vi "Format Test Configurations.vi"(0 "Test Configuration":T3(array[cluster]) {"Test Ranking" items=["Low", "Normal", "High"]}) -> (4 "formatted string":string)   [LabVIEW 2020]
uses:
  <vilib>/addons/analyzer/_analyzerctrls.llb/VIAnCtl TestRanking.ctl
  <vilib>/addons/analyzer/_analyzerctrls.llb/VIAnCtl Config Control Value.ctl
  <vilib>/Utility/sysdir.llb/System Directory Type.ctl
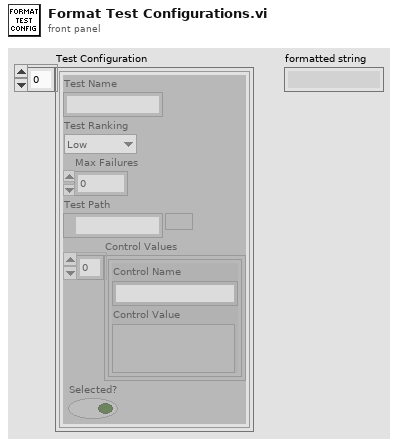
[diagram p1: front panel]
types:
  T1 = typedef "VIAnCtl TestRanking.ctl" = u16
  T2 = typedef "VIAnCtl Config Control Value.ctl" = cluster{"Control Name":string, "Control Value":variant}
  T3 = cluster{"Test Name":string, "Test Ranking":T1, "Max Failures":u32, "Test Path":path, "Control Values":T2[], "Selected?":bool}[]
  T4 = typedef "System Directory Type.ctl" = i32
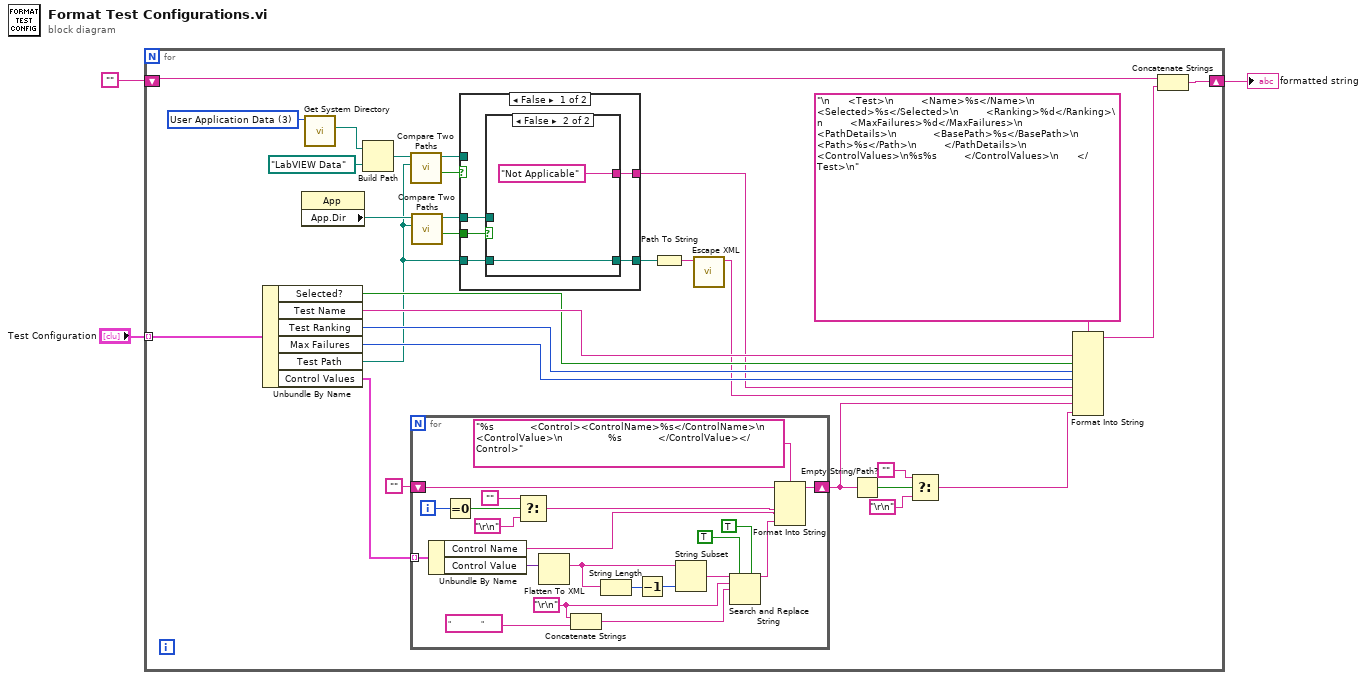
[diagram p0: block diagram]
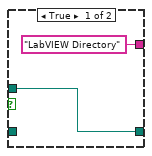
[diagram p2: hidden frame]
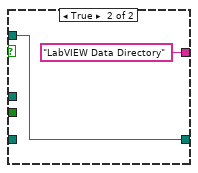
[diagram p3: hidden frame]
diagram:
  n1 = for {
    tunnel: "Test Configuration" -> [w33] mode=indexing
    shift-right: [w31] -> w1
    shift-left: "" -> [w32]
    w10 = T4 3 items=["User Home"=0, "User Desktop"=1, "User Documents"=2, "User Application Data"=3, "User Preferences"=4, "User Temporary"=5, "Public Documents"=6, "Public Application Data"=7, "Public Preferences"=8, "Public Cache"=13, "System Core Libraries"=9, "System Installed Libraries"=10, "Application Files"=11, "Boot Volume Root"=12] ("system directory type")
    n2 = Unbundle By Name(w33) -> ("Selected?"=w24:bool, "Test Name"=w30:string, "Test Ranking"=w28:T1, "Max Failures"=w27:u32, "Test Path"=w4:path, "Control Values"=w25:T2[])
    n3 = property class="App"() -> ("App.Dir"=w12:path)  [unwired: 2 in, 2 out]
    n4 = call <vilib>:"Get System Directory.vi"("system directory type"=w10) -> ("system directory"=w8:path)  [unwired: 10 in]
    n5 = Build Path(base path=w8, name or relative path=path "LabVIEW Data") -> (appended path=w7:path)
    n6 = call <vilib>:"Compare Two Paths.vi"("Path 2"=w4, "Path 1"=w7) -> ("Path 2 Relative to Path 1?"=w6:bool, "Relative Path from 1 to 2"=w5:path)  [unwired: 6 in, 2 out]
    n7 = for {
      tunnel: w25 -> [w65] mode=indexing
      shift-right: [w57] -> w20
      shift-left: "" -> [w58]
      i -> [w60]
      w53 = "\r\n"
      n8 = Unbundle By Name(w65) -> ("Control Name"=w45:string, "Control Value"=w64:variant)
      n9 = Equal To 0?(x=w60) -> (x = 0?=w63:bool)
      n10 = Select(t="", s=w63, f="\r\n") -> (s? t:f=w56:string)
      n11 = Flatten To XML(6:w64) -> (2:w49:string)
      n12 = Concatenate Strings(w53, "               ") -> (w52:string)
      n13 = String Length(string=w49) -> (length=w50:i32)
      n14 = Decrement(x=w50) -> (x-1=w48:i32)
      n15 = String Subset(string=w49, length (rest)=w48) -> (substring=w51:string)  [unwired: 1 in]
      n16 = Search and Replace String(replace all?=TRUE ("replace all? (F)"), multiline?=TRUE ("multiline? (F)"), input string=w51, search string=w53, replace string=w52) -> (result string=w46:string)  [unwired: 3 in, 3 out]
      n17 = Format Into String(format string="%s            <Control><ControlName>%s</ControlName>\n            <ControlValue>\n               %s            </ControlValue></Control>", initial string=w58, w56, w45, w46) -> (resulting string=w57:string)  [unwired: 1 in, 1 out]
    }
    n18 = call <vilib>:"Compare Two Paths.vi"("Path 2"=w4, "Path 1"=w12) -> ("Path 2 Relative to Path 1?"=w11:bool, "Relative Path from 1 to 2"=w16:path)  [unwired: 6 in, 2 out]
    n19 = case shown="False" w6 {
      tunnel: w16 -> [w38 _]
      tunnel: [w37 w44] -> w15
      tunnel: [w36 "LabVIEW Data Directory"] -> w13
      tunnel: w4 -> [w35 _]
      tunnel: w11 -> [w34 _]
      tunnel: w5 -> [_ w44]
      frame False {
        n20 = case shown="False" w34 {
          tunnel: w38 -> [w39 _]
          tunnel: w35 -> [_ w41]
          tunnel: ["LabVIEW Directory" "Not Applicable"] -> w36
          tunnel: [w39 w41] -> w37
          frame True {
          }
          frame False {
          }
        }
      }
      frame True {
      }
    }
    n21 = Path To String(path=w15) -> (string=w23:string)
    n22 = call <vilib>:"Escape XML.vi"("XML String In"=w23) -> ("XML String Out"=w14:string)  [unwired: 9 in, 1 out]
    n23 = Empty String/Path?(string/path=w20) -> (empty?=w21:bool)
    n24 = Select(t="", s=w21, f="\r\n") -> (s? t:f=w19:string)
    n25 = Format Into String(format string="\n      <Test>\n         <Name>%s</Name>\n         <Selected>%s</Selected>\n         <Ranking>%d</Ranking>\n         <MaxFailures>%d</MaxFailures>\n         <PathDetails>\n            <BasePath>%s</BasePath>\n            <Path>%s</Path>\n         </PathDetails>\n         <ControlValues>\n%s%s         </ControlValues>\n      </Test>\n", w30, w24, w28, w27, w13, w14, w20, w19) -> (resulting string=w26:string)  [unwired: 2 in, 1 out]
    n26 = Concatenate Strings(w32, w26) -> (w31:string)
  }
  "formatted string" <- w1
